vi "Spectrometer_scan wavelength_1 lockin_1_good_#.vi"() -> ()   [LabVIEW 2011]
uses:
  <vilib>/Utility/file.llb/Write To Spreadsheet File (DBL).vi
panel:
  out "real Wavelength":dbl=571.998 format="%.2f"
  in  "XSpectraSense":refnum<k7>(container)
  in  "Tab Control":enum32{"Spectrometer", "Lockin 2", "Save data"}(tab)=enum."Save data"
  out "step #":i32=20
  out "N":dbl=20.0
  in  "step size(nm)":dbl=0.1
  in  "fianl wavelength":dbl=572.0
  in  "initial wavelength":dbl=570.0
  out "SpectraHub output":dbl
  in  "data interval  time(ms)":dbl=1200.0
  out "?":bool=TRUE
  in  "Ready To Go? 5":bool
  in  "Sensitivity Range 2":u8(ring)=23 items=["2nV", "2nV", "5nV", "10nV", "20nV", "50nV", "100nV", "200nV", "500nV", "1µV", "2µV", "5µV", "10µV", "20µV", "50µV", "100µV", "200µV", "500µV", "1mV", "2mV", "5mV", "10mV", "20mV", "50mV", "100mV", "200mV", "500mV", "1V"]
  out "Units 2":string="mV"
  out "Display 2":dbl=0.01 format="%.3f"
  in  "Display Type 2":u16(ring)=2 items=["X %", "Y %", "X Calibrated", "Y Calibrated", "Mag %", "Mag Calibrated", "Phase Degrees", "Ratio", "Log Ratio", "ADC 1", "ADC 2", "ADC 3", "Noise %", "Noise Calibrated", "Ref Frequency", "Equation 1", "Equation 2"]
  in  "Input Mode  2":u16(ring)=1 items=["Inputs Grounded (test)", "A (Single-Ended Voltage)", "-B (Inverting Single Ended Voltage)", "A-B (Differential Voltage)", "B Current input - High Bandwidth", "B Current input - Low Noise"]
  in  "VISA session (for class) 2":refnum<visa-resource-name>="GPIB0::13::INSTR"
  out "?":bool=TRUE
  in  "Ready To Go?":bool
  out "?":bool
  in  "Ready To Go? 6":bool
  in  "Path":path=path "E:/1.Users/Zaeill Kim/2.Experiment/5.Data/1129'06_S4_wave dependence/TRFR_DAC_S4_pressure15_probe wavelength dependence1/570nm_minichrom set.txt"
  out "lockin 2 output":cluster{dbl[], dbl[]}(graph)={[569.999, 570.099, 570.198, 570.298, 570.399, 570.498, 570.598, 570.699, 570.797, 570.898, 570.998, 571.099, 571.197, 571.298, 571.399, 571.499, 571.598, 571.698, 571.799, 571.897, 571.998], [0.19, 0.25, 0.665, 2.32, 7.97, 20.97, 39.11, 54.455, 59.61, 54.81, 43.49, 27.82, 12.74, 3.645, 0.585, 0.11, 0.05, 0.035, 0.025, 0.015, 0.01]}
  in  "Comments":string="\n"
  in  "stop":bool
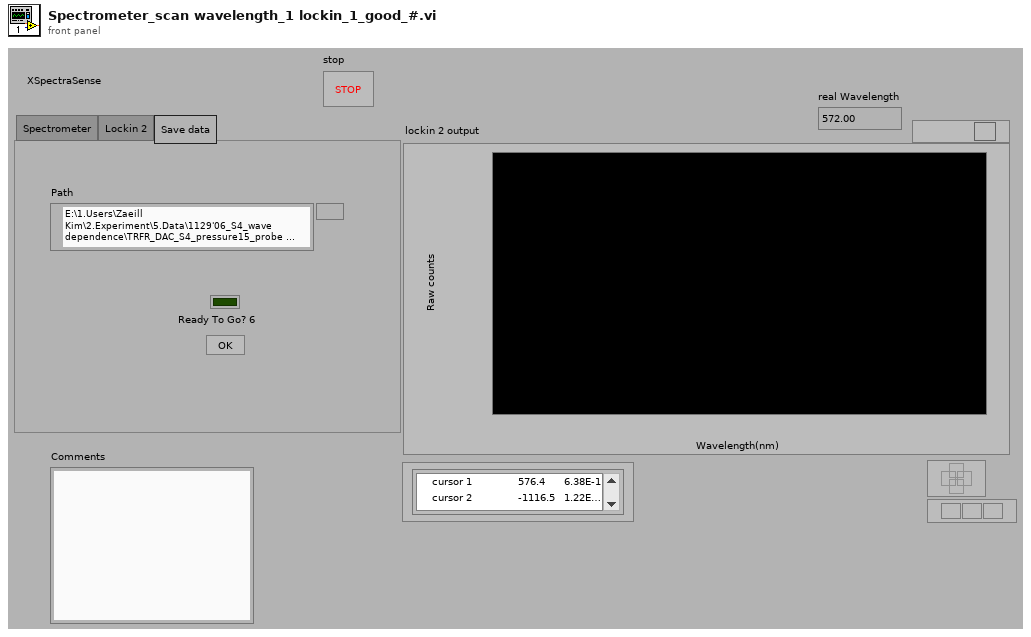
[diagram p1: front panel]
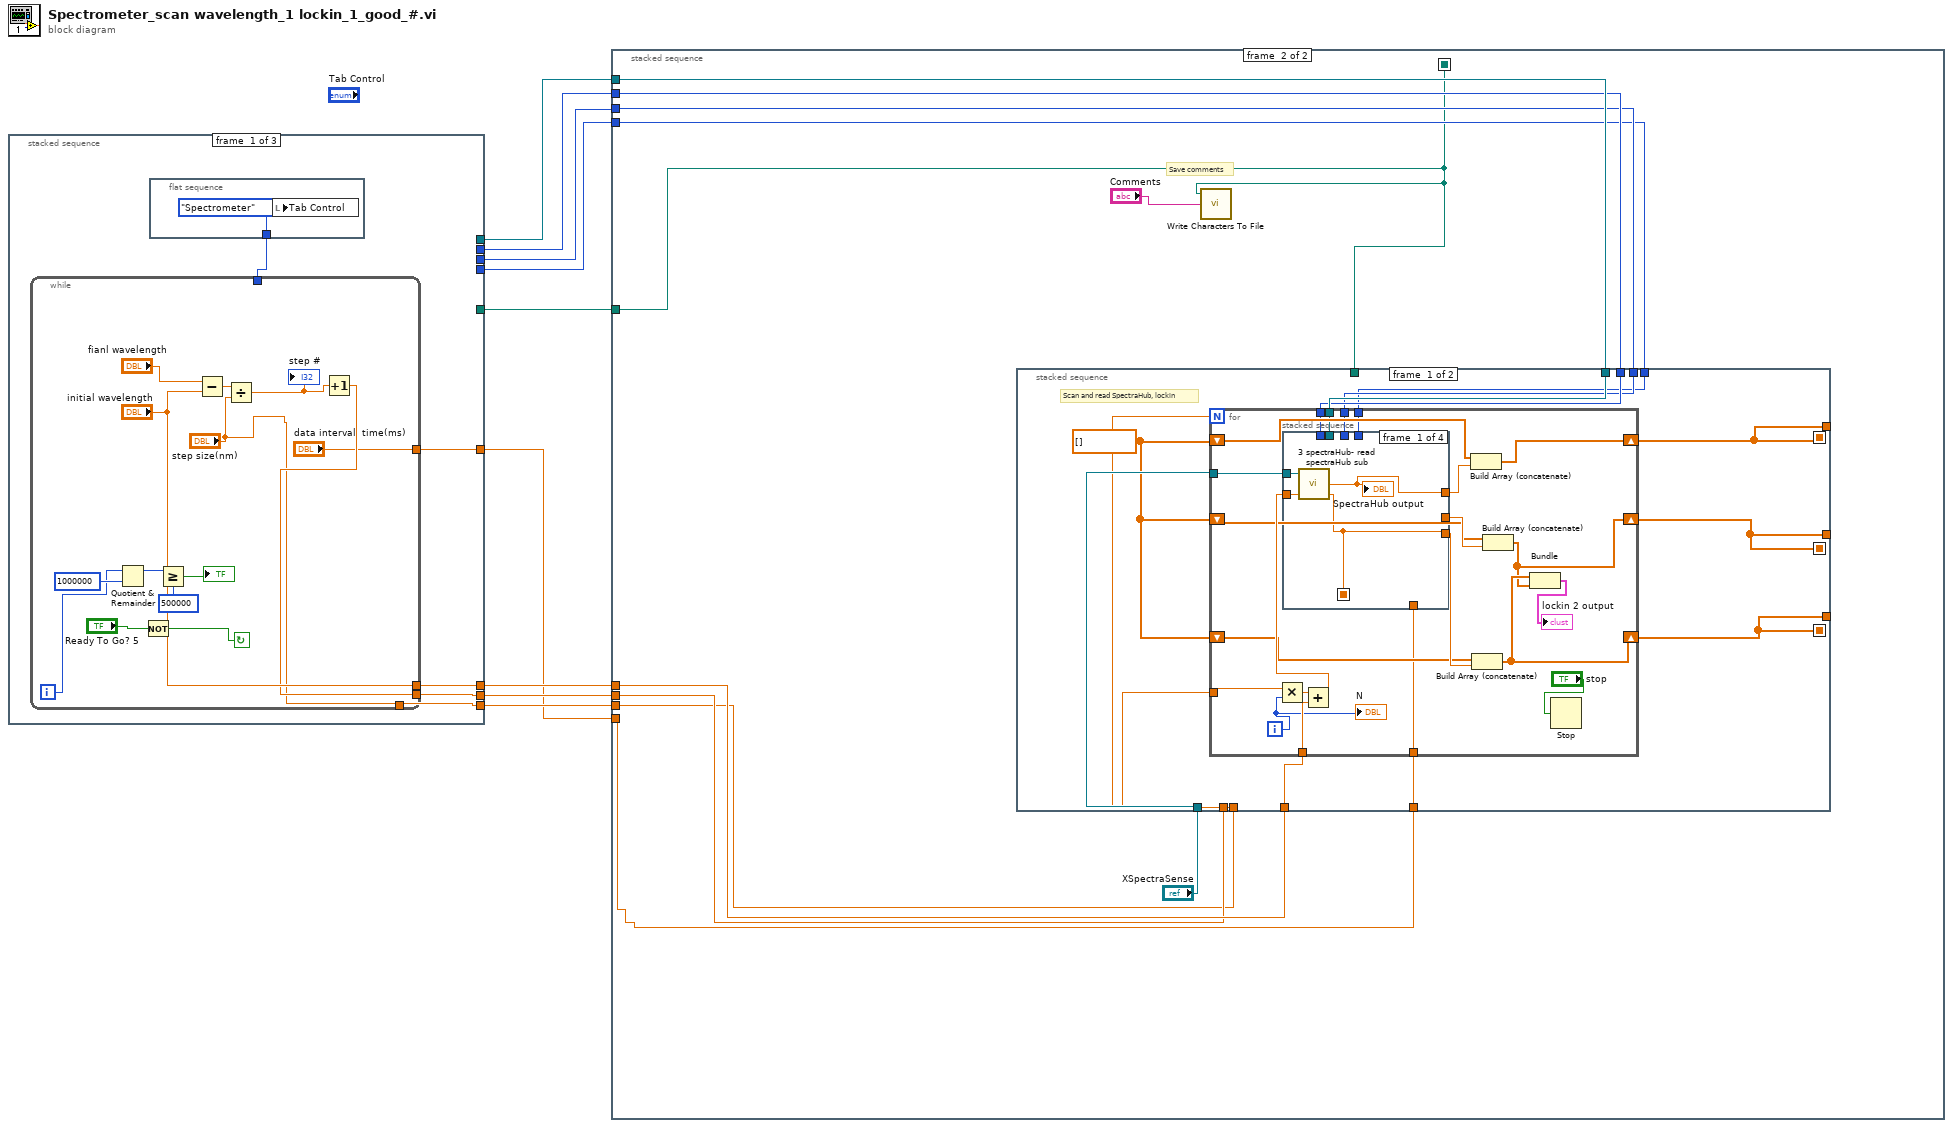
[diagram p0: block diagram]
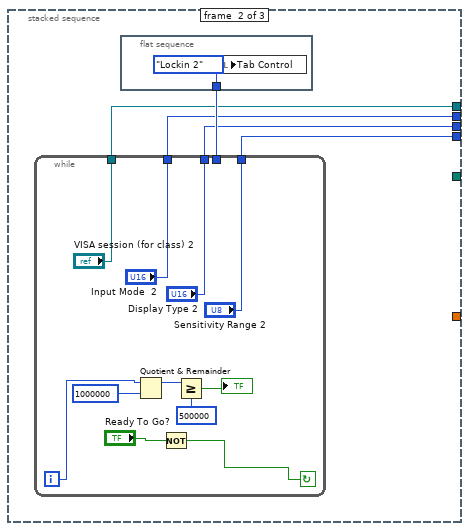
[diagram p2: hidden frame]
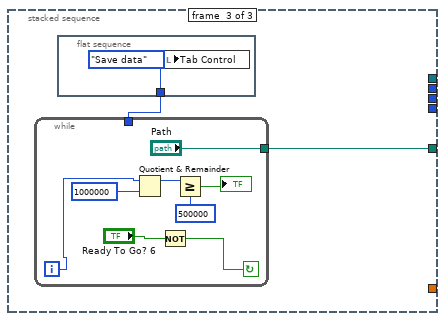
[diagram p3: hidden frame]
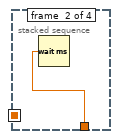
[diagram p5: hidden frame]
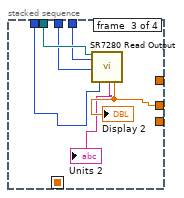
[diagram p6: hidden frame]
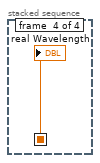
[diagram p7: hidden frame]
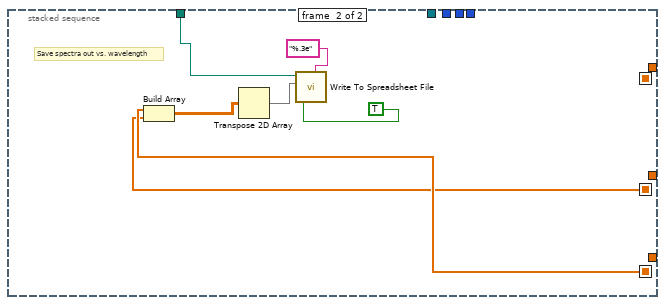
[diagram p8: hidden frame]
diagram:
  n1 = stacked-sequence {
    tunnel: [w14 _ _] -> w9
    tunnel: [w13 _ _] -> w8
    tunnel: [w12 _ _] -> w7
    tunnel: [_ w33 _] -> w6
    tunnel: [_ w32 _] -> w5
    tunnel: [_ w31 _] -> w4
    tunnel: [_ w30 _] -> w3
    tunnel: [_ _ w48] -> w2
    tunnel: [w10 _ _] -> w1
    frame #0 {
      n2 = while {
        tunnel: ["initial wavelength"] -> w14
        tunnel: [w17] -> w13
        tunnel: ["step size(nm)"] -> w12
        tunnel: w11 -> [_]
        tunnel: ["data interval  time(ms)"] -> w10
        i -> [w19]
        stop <- w20 continue-if-true
        n3 = Quotient & Remainder(x=w19, y=1000000) -> (x-y*floor(x/y)=w23:i32)  [unwired: 1 out]
        n4 = Not(x="Ready To Go? 5") -> (.not. x?=w20:bool)
        n5 = Greater Or Equal?(x=w23, y=500000) -> (x >= y?=→"?":bool)
        n6 = Subtract(x="fianl wavelength", y="initial wavelength") -> (x-y=w28:dbl)
        n7 = Divide(x=w28, y="step size(nm)") -> (x/y=w18:dbl)
        "step #" <- w18
        n8 = Increment(x=w18) -> (x+1=w17:dbl)
      }
      n9 = flat-sequence {
        tunnel: [w29] -> w11
        frame #0 {
          w29 = enum32{"Spectrometer", "Lockin 2", "Save data"}."Spectrometer" ("Tab Control")
          n10 = local write "Tab Control"(w29) -> ()
        }
      }
    }
    frame #1 {
      n11 = while {
        tunnel: w34 -> [_]
        tunnel: ["VISA session (for class) 2"] -> w33
        tunnel: ["Input Mode  2"] -> w32
        tunnel: ["Display Type 2"] -> w31
        tunnel: ["Sensitivity Range 2"] -> w30
        i -> [w39]
        stop <- w40 continue-if-true
        n12 = Quotient & Remainder(x=w39, y=1000000) -> (x-y*floor(x/y)=w43:i32)  [unwired: 1 out]
        n13 = Not(x="Ready To Go?") -> (.not. x?=w40:bool)
        n14 = Greater Or Equal?(x=w43, y=500000) -> (x >= y?=→"?":bool)
      }
      n15 = flat-sequence {
        tunnel: [w46] -> w34
        frame #0 {
          w46 = enum32{"Spectrometer", "Lockin 2", "Save data"}."Lockin 2" ("Tab Control")
          n16 = local write "Tab Control"(w46) -> ()
        }
      }
    }
    frame #2 {
      n17 = while {
        tunnel: ["Path"] -> w48
        tunnel: w47 -> [_]
        i -> [w49]
        stop <- w50 continue-if-true
        n18 = Quotient & Remainder(x=w49, y=1000000) -> (x-y*floor(x/y)=w53:i32)  [unwired: 1 out]
        n19 = Not(x="Ready To Go? 6") -> (.not. x?=w50:bool)
        n20 = Greater Or Equal?(x=w53, y=500000) -> (x >= y?=→"?":bool)
      }
      n21 = flat-sequence {
        tunnel: [w57] -> w47
        frame #0 {
          w57 = enum32{"Spectrometer", "Lockin 2", "Save data"}."Save data" ("Tab Control")
          n22 = local write "Tab Control"(w57) -> ()
        }
      }
    }
  }
  n23 = stacked-sequence {
    seq-local: [_ w59] -> [_ _]
    tunnel: w9 -> [_ w66]
    tunnel: w8 -> [_ w65]
    tunnel: w7 -> [_ w64]
    tunnel: w6 -> [_ w63]
    tunnel: w5 -> [_ w62]
    tunnel: w4 -> [_ w61]
    tunnel: w3 -> [_ w60]
    tunnel: w2 -> [_ w59]
    tunnel: w1 -> [_ w58]
    frame #0 {
    }
    frame #1 {
      # "Save comments"
      n24 = stacked-sequence {
        seq-local: [w77 _] -> [_ _]
        seq-local: [w76 _] -> [_ w122]
        seq-local: [w70 _] -> [_ w117]
        tunnel: "XSpectraSense" -> [w81 _]
        tunnel: w65 -> [w78 _]
        tunnel: w66 -> [w80 _]
        tunnel: w64 -> [w79 _]
        tunnel: [w77 _] -> _
        tunnel: [w76 _] -> _
        tunnel: w59 -> [_ w118]
        tunnel: w63 -> [w75 _]
        tunnel: w62 -> [w74 _]
        tunnel: w61 -> [w73 _]
        tunnel: w60 -> [w72 _]
        tunnel: [w70 _] -> _
        tunnel: w58 -> [w69 _]
        frame #0 {
          w71 = dbl[] []
          # "Scan and read SpectraHub, lockin"
          n25 = for {
            N: w78 -> [_]
            tunnel: w81 -> [w103]
            tunnel: w80 -> [w102]
            tunnel: w79 -> [w93]
            shift-right: [w97] -> w77
            shift-left: w71 -> [w99]
            shift-right: [w85] -> w76
            shift-left: w71 -> [w95]
            tunnel: w75 -> [w92]
            tunnel: w74 -> [w91]
            tunnel: w73 -> [w90]
            tunnel: w72 -> [w89]
            shift-right: [w84] -> w70
            shift-left: w71 -> [w86]
            tunnel: w69 -> [w82]
            i -> [w94]
            n26 = Multiply(x=w93, y=w94) -> (x*y=w101:dbl)
            n27 = Add(x=w101, y=w102) -> (x+y=w100:dbl)
            n28 = stacked-sequence {
              seq-local: [w104 _ _ _] -> [_ _ _ w115]
              tunnel: w103 -> [w107 _ _ _]
              tunnel: w100 -> [w106 _ _ _]
              tunnel: [w105 _ _ _] -> w88
              tunnel: [w104 _ _ _] -> w98
              tunnel: w92 -> [_ _ w114 _]
              tunnel: w91 -> [_ _ w111 _]
              tunnel: w90 -> [_ _ w112 _]
              tunnel: w89 -> [_ _ w113 _]
              tunnel: [_ _ w110 _] -> w87
              tunnel: w82 -> [_ w108 _ _]
              frame #0 {
                n29 = call "3 spectraHub- read spectraHub sub.vi"("Goto  wavelength"=w106, "XSpectraSense"=w107) -> ("real Wavelength"=w104:dbl, "SpectraHub output"=w105:dbl)  [unwired: 1 in, 1 out]
                "SpectraHub output" <- w105
              }
              frame #1 {
                n30 = Wait (ms)(milliseconds to wait=w108) -> ()  [unwired: 1 out]
              }
              frame #2 {
                n31 = call "SR7280 Read Output.vi"("VISA session (for class)"=w114, "Range"=w113, "Display Type"=w112, "Input Mode"=w111) -> ("Units"=→"Units 2":string, "Display"=w110:dbl)  [unwired: 7 in, 7 out]
                "Display 2" <- w110
              }
              frame #3 {
                "real Wavelength" <- w115
              }
            }
            n32 = Build Array (concatenate)(w99, w88) -> (w97:dbl[])
            n33 = Build Array (concatenate)(w95, w98) -> (w85:dbl[])
            n34 = Build Array (concatenate)(w86, w87) -> (w84:dbl[])
            n35 = Bundle(w85, w84) -> (→"lockin 2 output":cluster{dbl[], dbl[]})  [unwired: 1 in]
            n36 = Stop(stop? (T)="stop") -> ()
            "N" <- w94
          }
        }
        frame #1 {
          # "Save spectra out vs. wavelength"
          n37 = Build Array(w122, w117) -> (w121:dbl[][])
          n38 = Transpose 2D Array(2D array=w121) -> (transposed array=w120:dbl[][])
          n39 = call-poly <vilib>:"Write To Spreadsheet File.vi"("format (%.3f)"="%.3e", "append to file? (new file:F)"=TRUE, "2D data"=w120, "file path (dialog if empty)"=w118) -> ()  [unwired: 4 in, 1 out]
        }
      }
      n40 = call <vilib>:"Write Characters To File.vi"("character string"="Comments", "file path (dialog if empty)"=w59) -> ()  [unwired: 3 in, 1 out]
    }
  }
